vi "System Semaphore Release.vi"(8 "error in (no error)":errorcluster, 11 "SemaphoreHandle":u16 format="%.0x") -> (0 "error out":errorcluster, 3 "PreviousCount":i32)   [LabVIEW 2011]
uses:
  kernel32.dll
panel:
  in  "PreviousCount in":i32
  # "Releases System Semaphore by Handle\n(Increases Count by 1)"
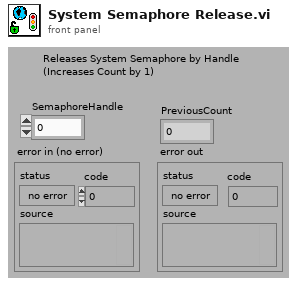
[diagram p1: front panel]
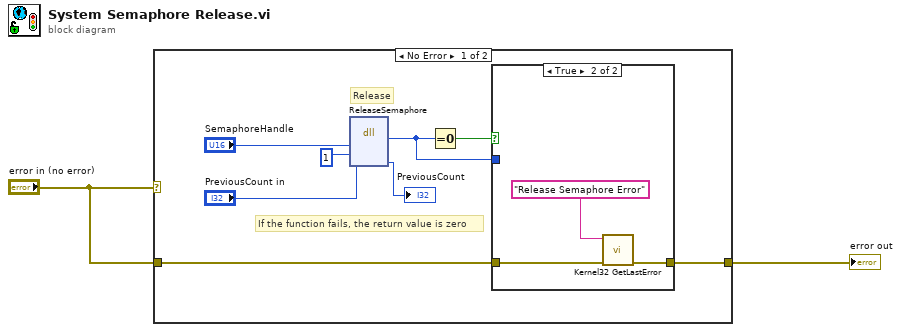
[diagram p0: block diagram]
diagram:
  n1 = case shown="No Error" "error in (no error)" {
    tunnel: "error in (no error)" -> [w5 w15]
    tunnel: [w4 w15] -> w2
    frame No Error {
      # "If the function fails, the return value is zero"
      # "Release"
      n2 = dll-call lib="kernel32.dll" fn="ReleaseSemaphore"("SemaphoreHandle"="SemaphoreHandle", "ReleaseCount"=1, "PreviousCount"="PreviousCount in") -> (w3:u8, "PreviousCount"=→"PreviousCount":i32)  [unwired: 5 in, 2 out]
      n3 = Equal To 0?(x=w3) -> (x = 0?=w6:bool)
      n4 = case shown="True" w6 {
        tunnel: w5 -> [w11 w14]
        tunnel: [w11 w13] -> w4
        tunnel: w3 -> [_ _]
        frame False {
          # "No Error"
        }
        frame True {
          n5 = call "Kernel32 GetLastError.vi"("error in (no error)"=w14, "Message"="Release Semaphore Error" ("source")) -> ("error out"=w13:errorcluster)  [unwired: 9 in]
        }
      }
    }
    frame Error {
    }
  }
  "error out" <- w2
